vi "Main.vi"(11 "Module Admin":refnum<class "Delacor_lib_QMH_Module Admin.lvclass">) -> ()   [LabVIEW 2020, in "Config.lvlib"]
doc: "This template is based off of the Queued Message Handler design pattern and the Queued Message Handler project template that ships with LabVIEW.\n\nThe main difference is that the queue is private to this module and communication between modules is performed via Broadcast and Request events.\n\nRequest events are wrapped in public API methods and are handled in the Event Handling Loop (EHL) of this VI. Any module can register for Broadcast events sent by this module. The EHL generates messages based on user interface actions.\n\nThe Message Handling Loop (MHL) processes messages generated by the EHL, or by other messages. The messages are string values, so new messages can be added easily to the Message Cases case structure in the MHL. Each message cluster can also provide an optional value for Message Data, which is a variant that can be converted to whatever message-specific data is required.\n_____\nBased on Delacor QMH Project Template 5.0.0.82."
uses:
  Config.lvlib
  <vilib>/Delacor/Delacor QMH/Libraries/Module Admin_class/Delacor_lib_QMH_Module Admin.lvclass
  Module Data--cluster.ctl
  Stop Argument--cluster.ctl
  <vilib>/Delacor/Delacor QMH/Libraries/Message Queue_class/Delacor_lib_QMH_Message Queue.lvclass/Delacor_lib_QMH_Message Queue.ctl
  <vilib>/Utility/miscctls.llb/LVPointTypeDef.ctl
  <vilib>/Delacor/Delacor QMH/Libraries/Module Admin_class/Delacor_lib_QMH_Module Admin.lvclass/Delacor_lib_QMH_Module Admin.ctl
  <vilib>/Delacor/Delacor QMH/Libraries/Message Queue_class/Delacor_lib_QMH_Enqueue Message (Single).vi
  <vilib>/Delacor/Delacor QMH/Libraries/Module Admin_class/Delacor_lib_QMH_Get External Launch.vi
  <vilib>/Utility/error.llb/Error Cluster From Error Code.vi
  <vilib>/ErrorRing/Error Ring.xnode
  <vilib>/Delacor/Delacor QMH/Libraries/Message Queue_class/Delacor_lib_QMH_Message Queue.lvclass
  Coins/Coins.lvlib
panel:
  in  "Coins":cluster{"Numeric":dbl, "Boolean Text":string}[](array[cluster])
  out "error out":errorcluster
  out "Status":string
  # "Config"
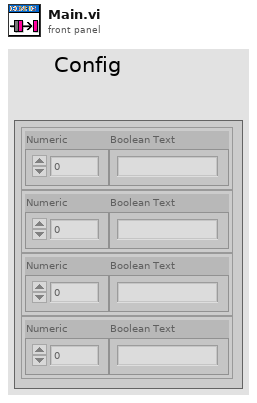
[diagram p1: front panel]
types:
  T1 = typedef "Config.lvlib/Request Events--cluster.ctl" = cluster{"Stop Module":refnum<user-event>, "Show Panel":refnum<user-event>, "Hide Panel":refnum<user-event>, "Get Module Execution Status":refnum<user-event>, "Show Diagram":refnum<user-event>}
  T2 = typedef "Config.lvlib/Module Data--cluster.ctl" = cluster{"Status":string}
  T3 = enum32{"invalid lock state", "Not Locked", "Locked (No Password)", "Password-protected"}
  T4 = typedef "Config.lvlib/Stop Argument--cluster.ctl" = cluster{"Origin":string, "Exit via Stop Module Req?":bool, "Wait for Module to stop?":bool}
  T5 = typedef "LVPointTypeDef.ctl" = cluster{"Horizontal":i16, "Vertical":i16}
  T6 = enum32{"Invalid", "Standard", "Closed", "Hidden", "Minimized", "Maximized"}
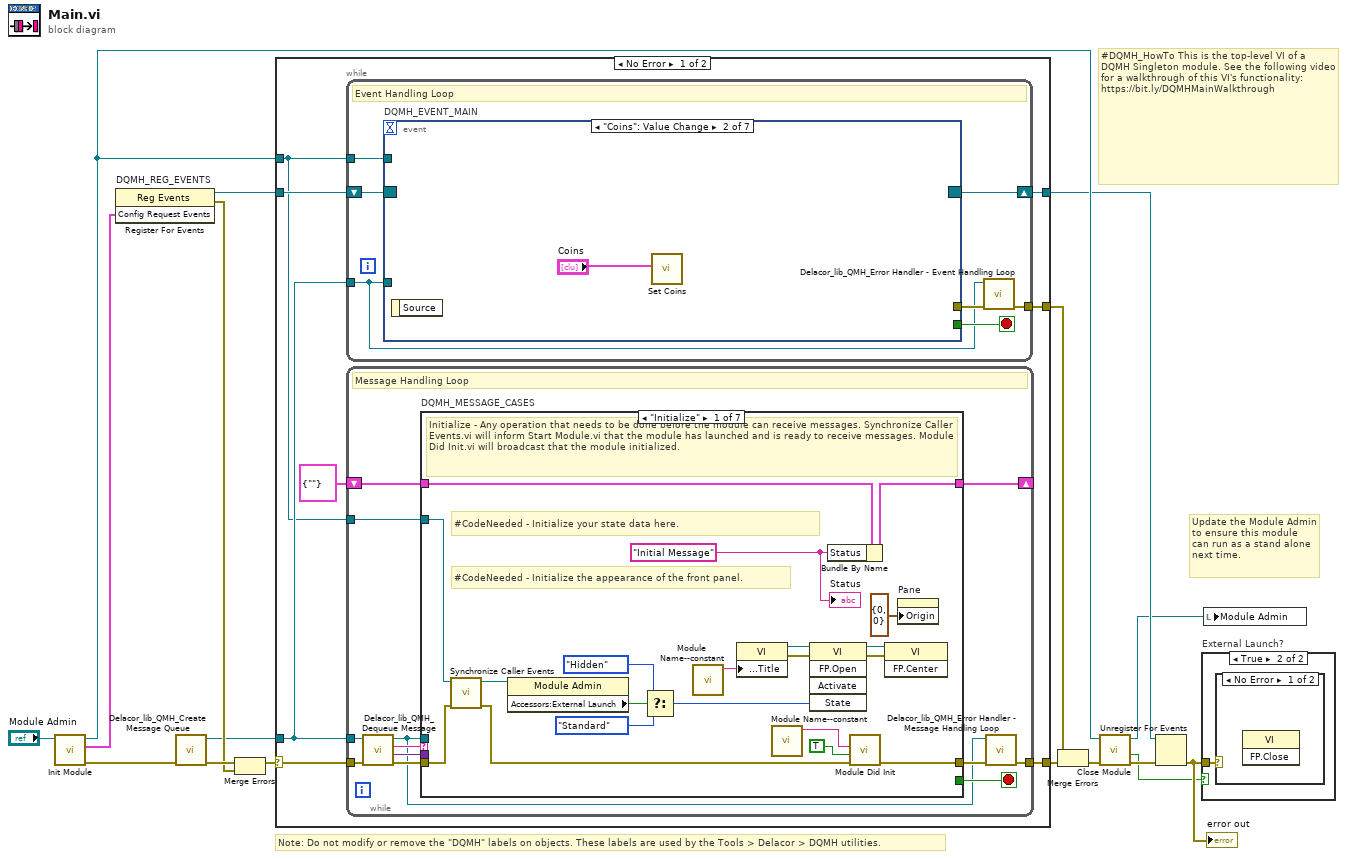
[diagram p0: block diagram]
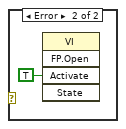
[diagram p3: hidden frame]
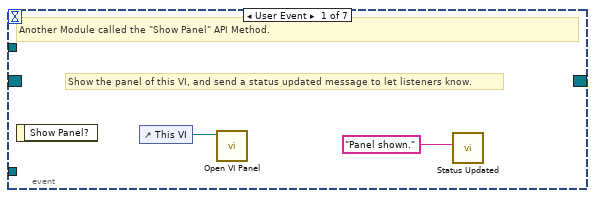
[diagram p4: hidden frame]
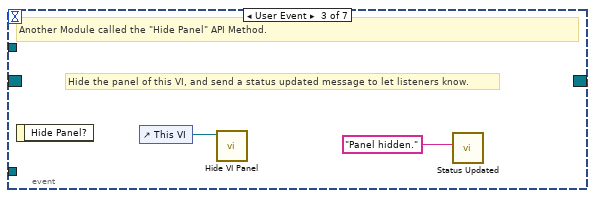
[diagram p5: hidden frame]
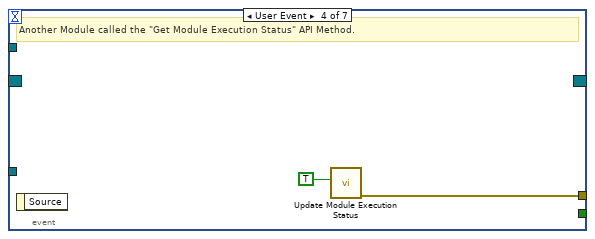
[diagram p6: hidden frame]
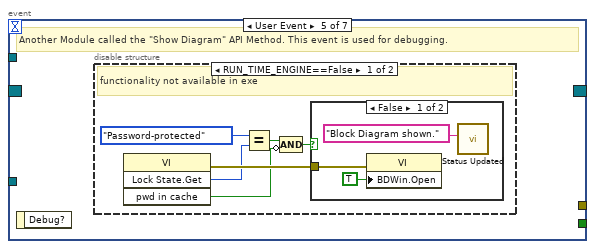
[diagram p7: hidden frame]
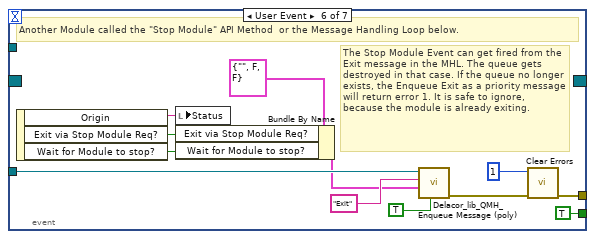
[diagram p10: hidden frame]
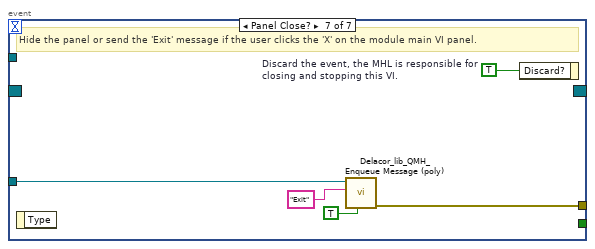
[diagram p11: hidden frame]
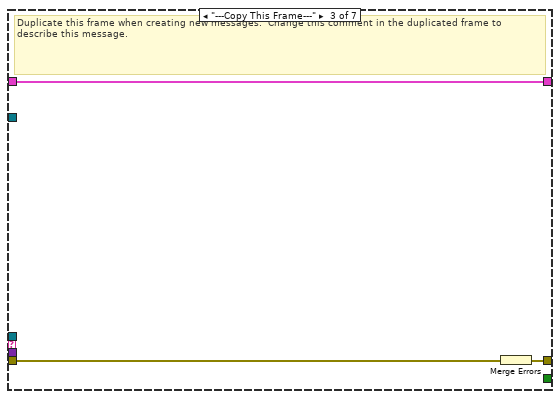
[diagram p13: hidden frame]
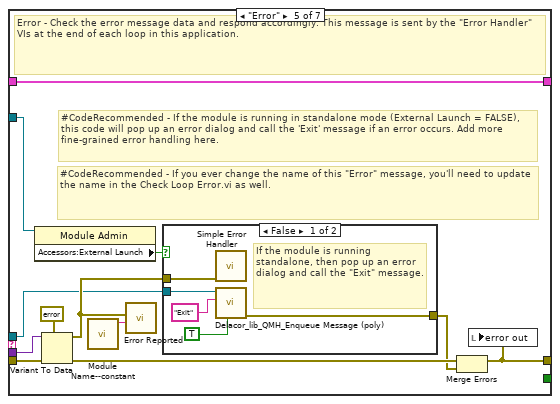
[diagram p15: hidden frame]
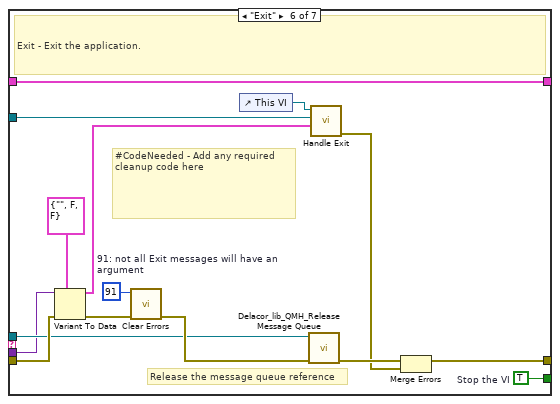
[diagram p17: hidden frame]
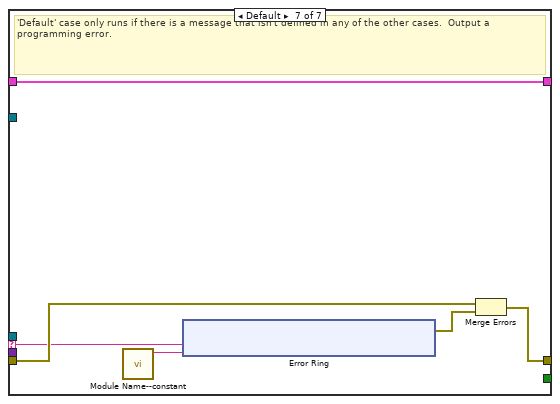
[diagram p18: hidden frame]
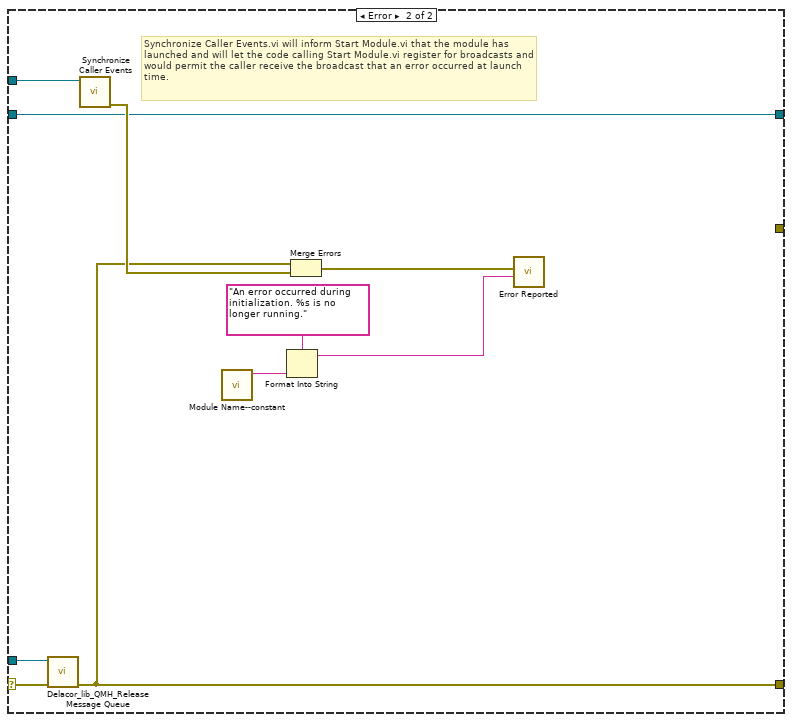
[diagram p19: hidden frame]
diagram:
  # "#DQMH_HowTo This is the top-level VI of a DQMH Singleton module. See the following video for a walkthrough of this VI's functionality: https://bit.ly/DQMHMainWalkthrough"
  # "Note: Do not modify or remove the \"DQMH\" labels on objects. These labels are used by the Tools > Delacor > DQMH utilities."
  # "Update the Module Admin to ensure this module can run as a stand alone next time."
  n1 = call "Init Module.vi"("Singleton Module Admin in"="Module Admin") -> ("error out"=w16:errorcluster, "Config Request Events"=w5:T1, "Singleton Module Admin out"=w8:refnum<class "Delacor_lib_QMH_Module Admin.lvclass">)  [unwired: 8 in]
  n2 = register-events "DQMH_REG_EVENTS"(w5) -> (reference out=w6:refnum<event-registration>, error out=w9:errorcluster)  [unwired: 2 in]
  n3 = call <vilib>:"Delacor_lib_QMH_Create Message Queue.vi"("error in (no error)"=w16) -> ("error out"=w11:errorcluster, "Message Queue"=w4:refnum<class "Delacor_lib_QMH_Message Queue.lvclass">)  [unwired: 9 in]
  n4 = Merge Errors(w11, w9) -> (w10:errorcluster)
  n5 = case shown="No Error" w10 {
    selector: w10 -> [w23 w153]
    tunnel: [w25 w152] -> w17
    tunnel: [w22 w158] -> w7
    tunnel: w6 -> [w20 w158]
    tunnel: w4 -> [w19 w151]
    tunnel: [w24 _] -> w14
    tunnel: w8 -> [w18 w154]
    frame No Error {
      n6 = while {
        tunnel: w19 -> [w26]
        shift-right: [w29] -> w22
        shift-left: w20 -> [w30]
        tunnel: [w31] -> w24
        tunnel: w18 -> [w27]
        stop <- w28 stop-if-true
        # "Event Handling Loop"
        n7 = event "DQMH_EVENT_MAIN" shown="[1] \"Coins\": Value Change" {
          selector: w30 -> [_ _ _ _ _ _ _]
          dyn-events: [_ _ _ _ _ _ _] -> w29
          timeout: _ -> [_ _ _ _ _ _ _]
          tunnel: [_ _ _ _ _ TRUE ("Discard?") _] -> w28
          tunnel: w26 -> [_ _ _ _ _ w56 w63]
          tunnel: [_ _ _ w39 _ w59 w65] -> w32
          tunnel: w27 -> [_ _ _ _ _ _ _]
          event User Event {
            # "Show the panel of this VI, and send a status updated message to let listeners know."
            # "Another Module called the \"Show Panel\" API Method."
            n8 = event-data() -> ()  [unwired: 1 in, 1 out]
            n9 = control-ref of="This VI"() -> (w34:refnum<vi>)
            n10 = call "Open VI Panel.vi"("VI"=w34) -> ()  [unwired: 10 in, 1 out]
            n11 = call "Status Updated.vi"("Status"="Panel shown." ("format string")) -> ()  [unwired: 10 in, 1 out]
          }
          event "Coins": Value Change {
            n12 = event-data() -> ()  [unwired: 1 in, 1 out]
            n13 = call "Set Coins.vi"("Coins"="Coins") -> ()  [unwired: 10 in, 1 out]
          }
          event User Event {
            # "Hide the panel of this VI, and send a status updated message to let listeners know."
            # "Another Module called the \"Hide Panel\" API Method."
            n14 = event-data() -> ()  [unwired: 1 in, 1 out]
            n15 = control-ref of="This VI"() -> (w37:refnum<vi>)
            n16 = call "Hide VI Panel.vi"("VI"=w37) -> ()  [unwired: 10 in, 1 out]
            n17 = call "Status Updated.vi"("Status"="Panel hidden." ("format string")) -> ()  [unwired: 10 in, 1 out]
          }
          event User Event {
            # "Another Module called the \"Get Module Execution Status\" API Method."
            n18 = event-data() -> ()  [unwired: 1 in, 1 out]
            n19 = call "Update Module Execution Status.vi"("Running?"=TRUE) -> ("error out"=w39:errorcluster)  [unwired: 10 in]
          }
          event User Event {
            # "Another Module called the \"Show Diagram\" API Method. This event is used for debugging."
            n20 = event-data() -> ()  [unwired: 1 in, 1 out]
            n21 = disable-structure shown="RUN_TIME_ENGINE==False" {
              frame condition #0 (active) {
                # "functionality not available in exe"
                n22 = invoke class="VI" method="Lock State.Get"() -> (error out=w45:errorcluster, "Get Lock State"=w44:T3, "pwd in cache"=w41:bool)  [unwired: 4 in, 1 out]
                n23 = Equal?(x=T3."Password-protected", y=w44) -> (x = y?=w42:bool)
                n24 = Compound Arithmetic op=AND(w42, invert w41) -> (w40:bool)
                n25 = case shown="False" w40 {
                  tunnel: w45 -> [w48 _]
                  frame False {
                    n26 = property class="VI"(error in=w48, "BDWin.Open"=TRUE ("Block Diagram Window:Open")) -> ()  [unwired: 1 in, 2 out]
                    n27 = call "Status Updated.vi"("Status"="Block Diagram shown." ("format string")) -> ()  [unwired: 10 in, 1 out]
                  }
                  frame True {
                    # "Password-protected VI, and the password is not in the cache. Do not show the diagram."
                  }
                }
              }
              frame condition #1 {
              }
            }
          }
          event User Event {
            # "The Stop Module Event can get fired from the Exit message in the MHL. The queue gets destroyed in that case. If the queue no longer exists, the Enqueue Exit as a priority message will return error 1. It is safe to ignore, because the module is already exiting."
            # "Another Module called the \"Stop Module\" API Method  or the Message Handling Loop below."
            n28 = event-data() -> ("Origin"=w55:string, "Exit via Stop Module Req?"=w51:bool, "Wait for Module to stop?"=w50:bool)  [unwired: 1 in]
            n29 = local write "Status"(w55) -> ()
            n30 = Bundle By Name(cluster=T4 {"Origin"="", "Exit via Stop Module Req?"=FALSE, "Wait for Module to stop?"=FALSE} ("Stop Argument"), "Exit via Stop Module Req?"=w51, "Wait for Module to stop?"=w50) -> (w49:T4)
            n31 = call-poly <vilib>:"Delacor_lib_QMH_Enqueue Message (poly).vi"("Priority Message? (F)"=TRUE, "Message Data"=w49, "Message"="Exit", "Message Queue in"=w56) -> ("error out"=w60:errorcluster)  [unwired: 6 in, 1 out]
            n32 = call <vilib>:"Clear Errors.vi"("error in (no error)"=w60, "specific error code to clear (0: all)"=1) -> ("error out"=w59:errorcluster)  [unwired: 4 in, 1 out]
          }
          event Panel Close? {
            w64 = TRUE  # Discard the event, the MHL is responsible for closing and stopping this VI.
            # "Hide the panel or send the 'Exit' message if the user clicks the 'X' on the module main VI panel."
            n33 = event-data() -> ()  [unwired: 1 in, 1 out]
            n34 = call-poly <vilib>:"Delacor_lib_QMH_Enqueue Message (poly).vi"("Priority Message? (F)"=TRUE, "Message"="Exit", "Message Queue in"=w63) -> ("error out"=w65:errorcluster)  [unwired: 7 in, 1 out]
            n35 = event-data("Discard?"=w64) -> ()  [unwired: 1 in, 1 out]
          }
        }
        n36 = call-dynamic "Delacor_lib_QMH_Error Handler - Event Handling Loop.vi"("error in (no error)"=w32, "Message Queue in"=w26) -> ("dup error in"=w31:errorcluster)  [unwired: 8 in, 1 out]
      }
      n37 = while {
        tunnel: w19 -> [w68]
        shift-right: [w72] -> _
        shift-left: T2 {"Status"=""} ("Data Cluster") -> [w73]
        tunnel: w23 -> [w76]
        tunnel: [w74] -> w25
        tunnel: w18 -> [w66]
        stop <- w71 stop-if-true
        # "Message Handling Loop"
        n38 = call-dynamic "Delacor_lib_QMH_Dequeue Message.vi"("error in (no error)"=w76, "Message Queue in"=w68) -> ("error out"=w75:errorcluster, "Message Data"=w69:variant, "Message"=w70:string, "Message Queue out"=w67:refnum<class "Delacor_lib_QMH_Message Queue.lvclass">)  [unwired: 6 in]
        n39 = case "DQMH_MESSAGE_CASES" shown="\"Initialize\"" w70 {
          selector: w70 -> [_ _ _ _ _ _ w138]
          tunnel: w67 -> [_ _ _ _ w108 w130 _]
          tunnel: w75 -> [w95 w99 w102 w104 w115 w136 w140]
          tunnel: [w93 w99 w101 w104 w111 w133 w141] -> w77
          tunnel: w73 -> [w84 w98 w100 w103 w110 w129 w139]
          tunnel: [w83 w98 w100 w103 w110 w129 w139] -> w72
          tunnel: [_ _ _ _ _ w128 _] -> w71
          tunnel: w69 -> [_ _ _ _ w109 w127 _]
          tunnel: w66 -> [w85 _ _ _ w107 w122 _]
          frame "Initialize" {
            w78 = "Initial Message" ("Initial Message")
            # "#CodeNeeded - Initialize the appearance of the front panel."
            # "#CodeNeeded - Initialize your state data here."
            # "Initialize - Any operation that needs to be done before the module can receive messages. Synchronize Caller Events.vi will inform Start Module.vi that the module has launched and is ready to receive messages. Module Did Init.vi will broadcast that the module initialized."
            n40 = call "Synchronize Caller Events.vi"("error in (no error)"=w95, "Singleton Module Admin in"=w85) -> ("error out"=w94:errorcluster, "Singleton Module Admin out"=w80:refnum<class "Delacor_lib_QMH_Module Admin.lvclass">)  [unwired: 8 in]
            n41 = property class="Module Admin"(reference=w80) -> ("Accessors:External Launch"=w89:bool)  [unwired: 1 in, 2 out]
            n42 = Select(t=T6."Hidden" ("State"), s=w89, f=T6."Standard" ("State")) -> (s? t:f=w86:T6)
            n43 = call "Module Name--constant.vi"() -> ("Module Name"=w92:string)  [unwired: 11 in]
            n44 = property class="VI"("Front Panel.Title"=w92) -> (reference out=w91:refnum<vi>, error out=w97:errorcluster)  [unwired: 2 in]
            n45 = call "Module Name--constant.vi"() -> ("Module Name"=w81:string)  [unwired: 11 in]
            n46 = invoke class="VI" method="FP.Open"(reference=w91, error in=w97, "State"=w86) -> (reference out=w90:refnum<vi>, error out=w96:errorcluster)  [unwired: 2 in, 3 out]
            n47 = Bundle By Name(cluster=w84, "Status"=w78) -> (w83:T2)
            n48 = call "Module Did Init.vi"("error in (no error)"=w94, "Initialized?"=TRUE, "Origin"=w81) -> ("error out"=w93:errorcluster)  [unwired: 8 in]
            n49 = invoke class="VI" method="FP.Center"(reference=w90, error in=w96) -> ()  [unwired: 1 in, 3 out]
            n50 = property on="Pane" class="Pane"("Origin"=T5 {"Horizontal"=0, "Vertical"=0}) -> ()  [unwired: 2 in, 2 out]
            "Status" <- w78
          }
          frame "--- Module Specific ---" {
            # "Separator -- The following cases handle messages specific to this Module."
          }
          frame "---Copy This Frame---" {
            # "Duplicate this frame when creating new messages.  Change this comment in the duplicated frame to describe this message."
            n51 = Merge Errors(w102) -> (w101:errorcluster)
          }
          frame "--- Exit and Error Handling---" {
            # "Separator - The following cases handle errors and exit messages."
          }
          frame "Error" {
            # "#CodeRecommended - If you ever change the name of this \"Error\" message, you'll need to update the name in the Check Loop Error.vi as well."
            # "#CodeRecommended - If the module is running in standalone mode (External Launch = FALSE), this code will pop up an error dialog and call the 'Exit' message if an error occurs. Add more fine-grained error handling here."
            # "Error - Check the error message data and respond accordingly. This message is sent by the \"Error Handler\" VIs at the end of each loop in this application."
            n52 = property class="Module Admin"(reference=w107) -> ("Accessors:External Launch"=w106:bool)  [unwired: 1 in, 2 out]
            n53 = Variant To Data(error in=w115, type=errorcluster {"status"=FALSE, "code"=0, "source"=""} ("error constant"), Variant=w109) -> (data=w116:errorcluster, error out=w113:errorcluster)
            n54 = call "Module Name--constant.vi"() -> ("Module Name"=w105:string)  [unwired: 11 in]
            n55 = call "Error Reported.vi"("Additional Information"=w105, "Error"=w116) -> ()  [unwired: 9 in, 1 out]
            n56 = case shown="False" w106 {
              tunnel: [w121 _] -> w112
              tunnel: w108 -> [w119 _]
              tunnel: w116 -> [w120 _]
              frame False {
                # "If the module is running standalone, then pop up an error dialog and call the \"Exit\" message."
                n57 = call <vilib>:"Simple Error Handler.vi"("error in (no error)"=w120) -> ()  [unwired: 4 in, 5 out]
                n58 = call-poly <vilib>:"Delacor_lib_QMH_Enqueue Message (poly).vi"("Priority Message? (F)"=TRUE, "Message"="Exit", "Message Queue in"=w119) -> ("error out"=w121:errorcluster)  [unwired: 7 in, 1 out]
              }
              frame True {
                # "If the module was launched externally, calling the Error Reported broadcast VI is the only action performed by the \"Error\" message. The module's caller can then process the error appropriately."
              }
            }
            n59 = Merge Errors(w113, w112) -> (w111:errorcluster)
            n60 = local write "error out"(w111) -> ()
          }
          frame "Exit" {
            w126 = 91  # 91: not all Exit messages will have an argument
            w128 = TRUE  # Stop the VI
            # "Release the message queue reference"
            # "#CodeNeeded - Add any required cleanup code here"
            # "Exit - Exit the application."
            n61 = Variant To Data(error in=w136, type=T4 {"Origin"="", "Exit via Stop Module Req?"=FALSE, "Wait for Module to stop?"=FALSE} ("Stop Argument"), Variant=w127) -> (data=w124:T4, error out=w132:errorcluster)
            n62 = call <vilib>:"Clear Errors.vi"("error in (no error)"=w132, "specific error code to clear (0: all)"=w126) -> ("error out"=w135:errorcluster)  [unwired: 4 in, 1 out]
            n63 = control-ref of="This VI"() -> (w123:refnum<vi>)
            n64 = call-dynamic "Delacor_lib_QMH_Release Message Queue.vi"("error in (no error)"=w135, "Message Queue"=w130) -> ("error out"=w134:errorcluster)  [unwired: 9 in]
            n65 = call "Handle Exit.vi"("Stop Argument"=w124, "Admin in"=w122, "VI reference"=w123) -> ("error out"=w131:errorcluster)  [unwired: 7 in, 1 out]
            n66 = Merge Errors(w134, w131) -> (w133:errorcluster)
          }
          frame Default {
            # "'Default' case only runs if there is a message that isn't defined in any of the other cases.  Output a programming error."
            n67 = call "Module Name--constant.vi"() -> ("Module Name"=w137:string)  [unwired: 11 in]
            n68 = xnode "Error Ring"("parameter 0"=w138, "parameter 1"=w137) -> ("error out"=w142:errorcluster)
            n69 = Merge Errors(w140, w142) -> (w141:errorcluster)
          }
        }
        n70 = call-dynamic "Delacor_lib_QMH_Error Handler - Message Handling Loop.vi"("error in (no error)"=w77, "Message Queue in"=w67) -> ("dup error in"=w74:errorcluster)  [unwired: 8 in, 1 out]
      }
    }
    frame Error {
      # "Synchronize Caller Events.vi will inform Start Module.vi that the module has launched and will let the code calling Start Module.vi register for broadcasts and would permit the caller receive the broadcast that an error occurred at launch time."
      n71 = call-dynamic "Delacor_lib_QMH_Release Message Queue.vi"("error in (no error)"=w153, "Message Queue"=w151) -> ("error out"=w152:errorcluster)  [unwired: 9 in]
      n72 = call "Synchronize Caller Events.vi"("Singleton Module Admin in"=w154) -> ("error out"=w159:errorcluster)  [unwired: 9 in, 1 out]
      n73 = call "Module Name--constant.vi"() -> ("Module Name"=w157:string)  [unwired: 11 in]
      n74 = Format Into String(format string="An error occurred during initialization. %s is no longer running.", w157) -> (resulting string=w155:string)  [unwired: 2 in, 1 out]
      n75 = Merge Errors(w152, w159) -> (w160:errorcluster)
      n76 = call "Error Reported.vi"("Additional Information"=w155, "Error"=w160) -> ()  [unwired: 9 in, 1 out]
    }
  }
  n77 = Merge Errors(w14, w17) -> (w13:errorcluster)
  n78 = call "Close Module.vi"("error in (no error)"=w13, "Module Admin in"=w8) -> ("error out"=w15:errorcluster, "External Launch"=w1:bool, "Module Admin out"=w2:refnum<class "Delacor_lib_QMH_Module Admin.lvclass">)  [unwired: 7 in]
  n79 = Unregister For Events(event registration refnum=w7, error in=w15) -> (error out=w12:errorcluster)
  "error out" <- w12
  n80 = case "External Launch?" shown="True" w1 {
    tunnel: w12 -> [_ w161]
    frame False {
    }
    frame True {
      n81 = case shown="No Error" w161 {
        frame No Error {
          n82 = invoke class="VI" method="FP.Close"() -> ()  [unwired: 3 in, 3 out]
        }
        frame Error {
          n83 = invoke class="VI" method="FP.Open"("Activate"=TRUE ("Activate?")) -> ()  [unwired: 4 in, 5 out]
        }
      }
    }
  }
  n84 = local write "Module Admin"(w2) -> ()
